vi "Assert to Data Type.vi"(8 "error in (no error)":errorcluster, 11 "Assert":refnum<class "Assert.lvclass">) -> (0 "error out":errorcluster, 3 "Assert out":refnum<class "Assertion.lvclass">)   [LabVIEW 2017, in "Assertion.lvclass"]
uses:
  <vilib>/gpm_packages/@cs/data-type-serializer/source/Assertion/Assertion.lvclass
  <vilib>/gpm_packages/@cs/run-time-assertions/Source/Assert/Assert.lvclass
  <vilib>/gpm_packages/@cs/data-type-serializer/source/Assertion/Assertion.lvclass/Assertion.ctl
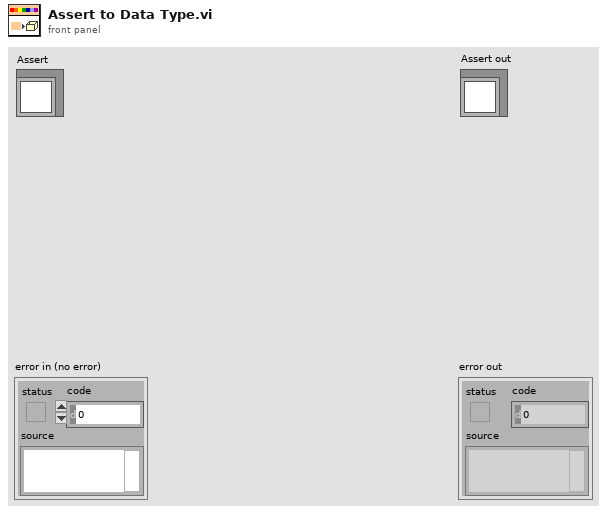
[diagram p1: front panel]
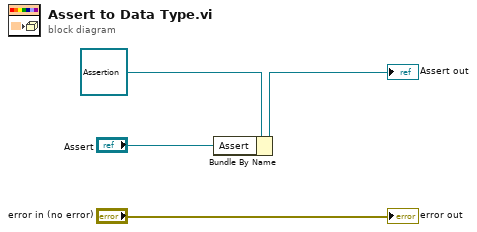
[diagram p0: block diagram]
diagram:
  n1 = Bundle By Name(cluster=refnum<class "Assertion.lvclass"> refnum ("Boolean in"), "Assert"="Assert") -> (→"Assert out":refnum<class "Assertion.lvclass">)
  "error out" <- "error in (no error)"
